vi "Get MCP Gain.vi"(11 "piGain":i32) -> (2 "function return":u32, 3 "piGain out":i32)   [LabVIEW 2018, in "Copy of Andor SDK.lvlib"]
doc: "EXPNETTYPE unsigned int WINAPI GetMCPGain(int * piGain);"
uses:
  Copy of Andor SDK.lvlib
  <userlib>/Andor SDK/ATMCD32D.dll
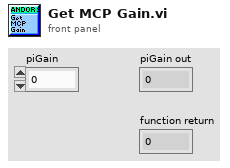
[diagram p1: front panel]
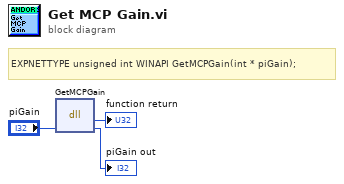
[diagram p0: block diagram]
diagram:
  # "EXPNETTYPE unsigned int WINAPI GetMCPGain(int * piGain);"
  n1 = dll-call lib="C:/Program Files (x86)/National Instruments/LabVIEW 2018/user.lib/Andor SDK/ATMCD32D.*" fn="GetMCPGain"("piGain"="piGain") -> (→"function return":u32, "piGain"=→"piGain out":i32)  [unwired: 3 in, 2 out]
